vi "直方图均衡化及累计结果.vi"() -> ()   [LabVIEW 2018]
uses:
  <vilib>/vision/NI_Vision_Development_Module.lvlib
panel:
  out "波形图 4":T1(graph)
  out "波形图 3":T1(graph)
  out "Image 2":T2(plugin-control)
  out "波形图 2":T1(graph)
  out "error out":errorcluster
  out "波形图":T1(graph)
  out "Image":T2(plugin-control)
  in  "路径":path
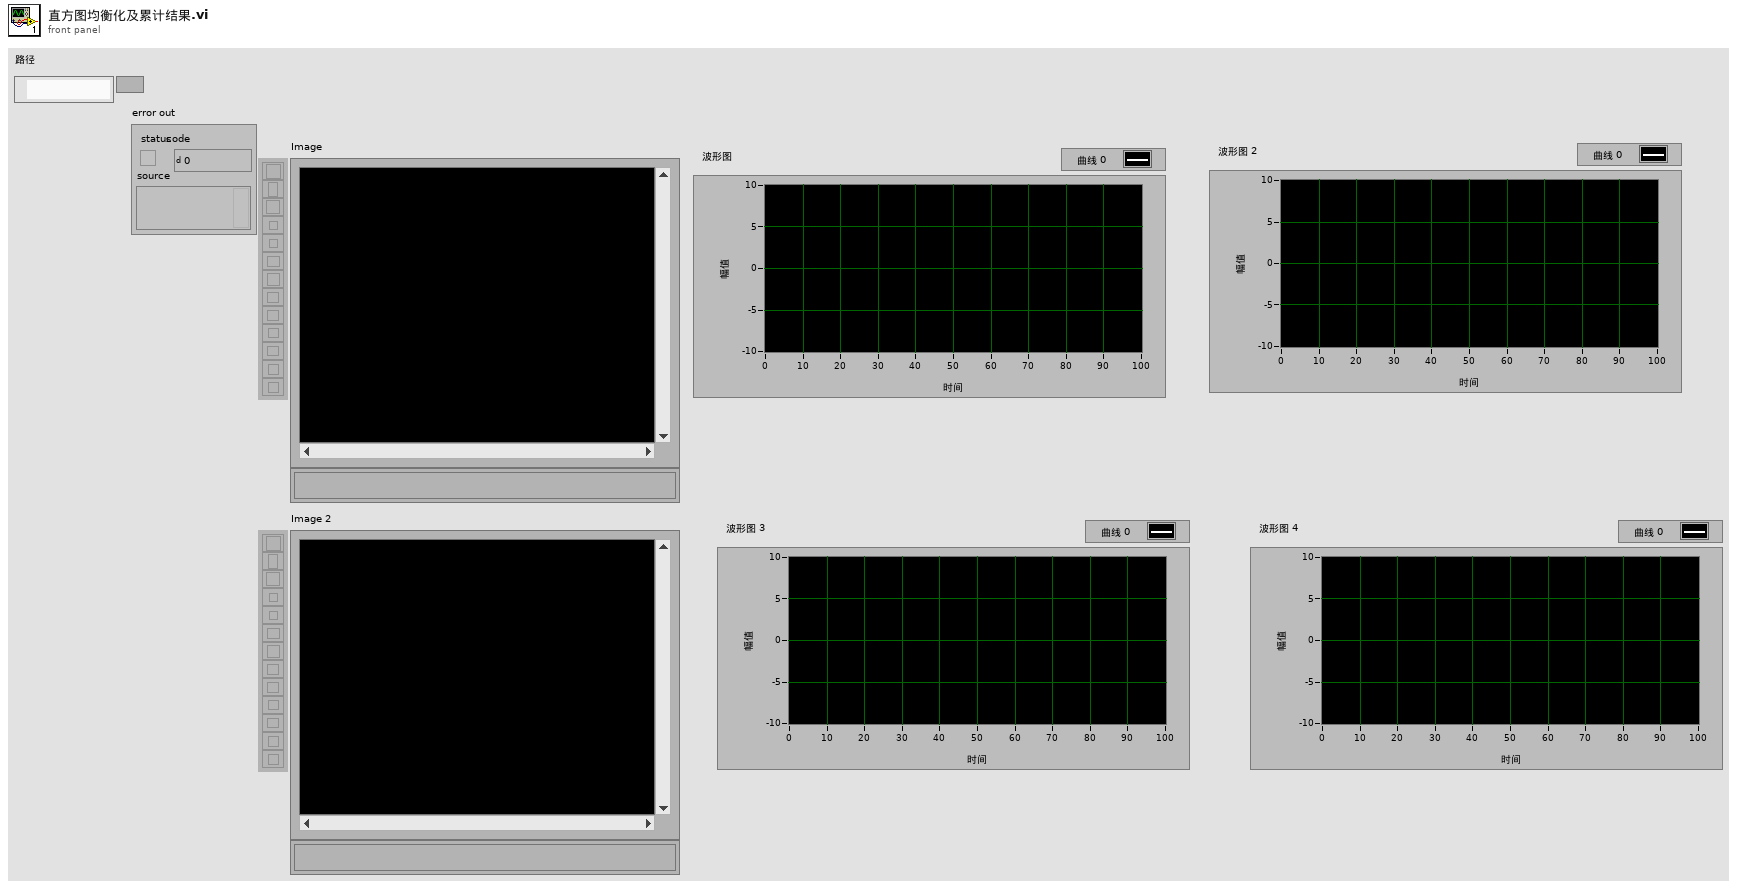
[diagram p1: front panel]
types:
  T1 = cluster{"Starting Value":sgl, "Incremental Value":sgl, "Histogram":u32[]}
  T2 = typedef "IMAQ Image.ctl" = refnum<image>
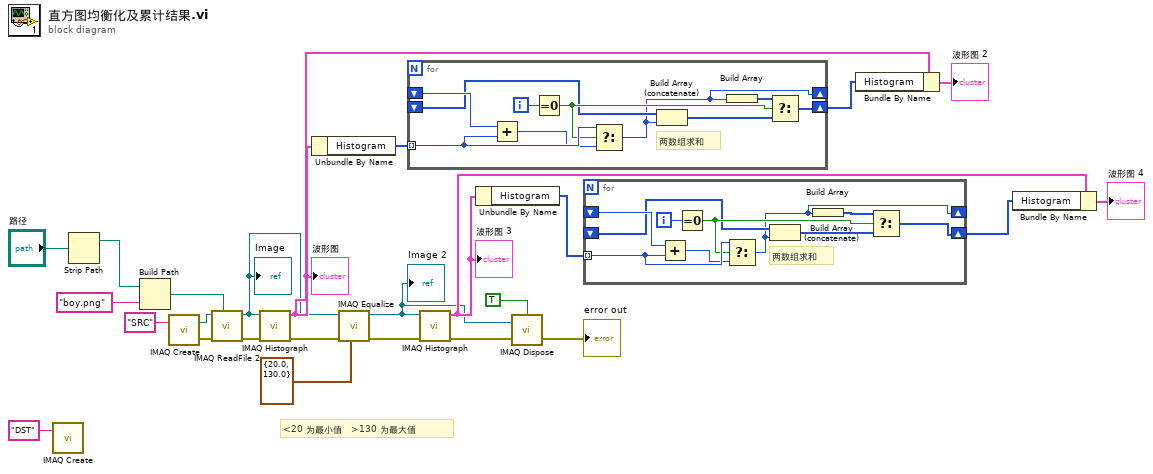
[diagram p0: block diagram]
diagram:
  # "<20 为最小值   >130 为最大值"
  n1 = call "IMAQ Create"("Image Name"="DST") -> ()  [unwired: 4 in, 2 out]
  n2 = Strip Path(path="路径") -> (stripped path=w24:path)  [unwired: 1 out]
  n3 = Build Path(base path=w24, name or relative path="boy.png" ("名称或相对路径")) -> (appended path=w20:path)
  n4 = call "IMAQ Create"("Image Name"="SRC") -> ("New Image"=w22:T2, "error out"=w21:errorcluster)  [unwired: 4 in]
  n5 = call "IMAQ ReadFile 2"("File Path"=w20, "error in (no error)"=w21, "Image"=w22) -> ("error out"=w18:errorcluster, "Image Out"=w10:T2)  [unwired: 4 in, 3 out]
  "Image" <- w10
  n6 = call "IMAQ Histograph"("error in (no error)"=w18, "Image"=w10) -> ("error out"=w9:errorcluster, "Histogram Graph"=w12:T1)  [unwired: 6 in, 2 out]
  "波形图" <- w12
  n7 = Unbundle By Name(w12) -> ("Histogram"=w14:u32[])
  n8 = call "IMAQ Equalize"("Range"=cluster{"Minimum":sgl, "Maximum":sgl} {"Minimum"=20.0, "Maximum"=130.0}, "error in (no error)"=w9, "Image Src"=w10) -> ("error out"=w7:errorcluster, "Image Dst Out"=w2:T2)  [unwired: 7 in]
  "Image 2" <- w2
  n9 = for {
    tunnel: w14 -> [w34] mode=indexing
    shift-right: [w27] -> _
    shift-left: _ -> [w35]
    shift-right: [w32] -> w13
    shift-left: _ -> [w28]
    i -> [w31]
    # "两数组求和"
    n10 = Add(x=w35, y=w34) -> (x+y=w33:u32)
    n11 = Equal To 0?(x=w31) -> (x = 0?=w29:bool)
    n12 = Select(t=w34, s=w29, f=w33) -> (s? t:f=w27:u32)
    n13 = Build Array (concatenate)(w28, w27) -> (w26:u32[])
    n14 = Build Array(w27) -> (w30:u32[])
    n15 = Select(t=w30, s=w29, f=w26) -> (s? t:f=w32:u32[])
  }
  n16 = call "IMAQ Histograph"("error in (no error)"=w7, "Image"=w2) -> ("error out"=w1:errorcluster, "Histogram Graph"=w5:T1)  [unwired: 6 in, 2 out]
  "波形图 3" <- w5
  n17 = Unbundle By Name(w5) -> ("Histogram"=w6:u32[])
  n18 = call "IMAQ Dispose"("All Images? (No)"=TRUE, "Image"=w2, "error in (no error)"=w1) -> ("error out"=→"error out":errorcluster)  [unwired: 3 in]
  n19 = for {
    tunnel: w6 -> [w44] mode=indexing
    shift-right: [w37] -> _
    shift-left: _ -> [w45]
    shift-right: [w42] -> w4
    shift-left: _ -> [w38]
    i -> [w41]
    # "两数组求和"
    n20 = Add(x=w45, y=w44) -> (x+y=w43:u32)
    n21 = Equal To 0?(x=w41) -> (x = 0?=w39:bool)
    n22 = Select(t=w44, s=w39, f=w43) -> (s? t:f=w37:u32)
    n23 = Build Array (concatenate)(w38, w37) -> (w36:u32[])
    n24 = Build Array(w37) -> (w40:u32[])
    n25 = Select(t=w40, s=w39, f=w36) -> (s? t:f=w42:u32[])
  }
  n26 = Bundle By Name(cluster=w12, "Histogram"=w13) -> (→"波形图 2":T1)
  n27 = Bundle By Name(cluster=w5, "Histogram"=w4) -> (→"波形图 4":T1)
